vi "Build Common Path Groups.vi"(8 "error in (no error)":errorcluster, 11 "File Group Paths":string[](array[string])) -> (0 "error out":errorcluster, 3 "Common Path map":map{string, string[]}(c390))   [LabVIEW 2019, in "Project.Dependencies Finder.lvlib" / "Dependency Source.lvclass"]
doc: "Order File Group paths in a map by the first folder name. \nThe file name is removed."
uses:
  Dependency Source.lvclass
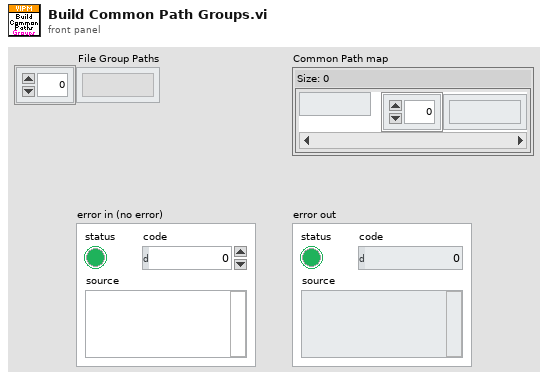
[diagram p1: front panel]
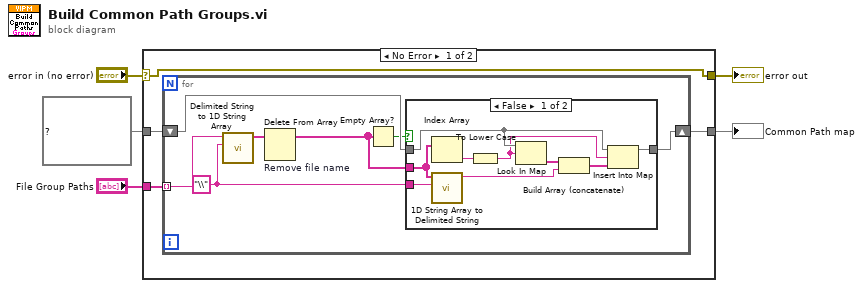
[diagram p0: block diagram]
diagram:
  n1 = case shown="No Error" "error in (no error)" {
    selector: "error in (no error)" -> [w6 w27]
    tunnel: [w6 w27] -> w3
    tunnel: [w9 w28] -> w4
    tunnel: map{string, string[]} {} ("map") -> [w8 w28]
    tunnel: "File Group Paths" -> [w7 _]
    frame No Error {
      n2 = for {
        shift-right: [w16] -> w9
        shift-left: w8 -> [w15]
        tunnel: w7 -> [w14] mode=indexing
        w12 = "\\" ("search string")
        n3 = call <vilib>:"Delimited String to 1D String Array.vi"("delimiter"=w12, "delimited string"=w14) -> ("string array"=w13:string[])  [unwired: 9 in]
        n4 = Delete From Array "Remove file name"(array=w13) -> (array with subset deleted=w11:string[])  [unwired: 2 in, 1 out]
        n5 = Empty Array?(array=w11) -> (empty?=w10:bool)
        n6 = case shown="False" w10 {
          tunnel: [w25 w26] -> w16
          tunnel: w15 -> [w24 w26]
          tunnel: w12 -> [w23 _]
          tunnel: w11 -> [w17 _]
          frame False {
            n7 = Index Array(array=w17) -> (element=w22:string)  [unwired: 1 in]
            n8 = call <vilib>:"1D String Array to Delimited String.vi"("delimiter"=w23, "string array"=w17) -> ("delimited string"=w19:string)  [unwired: 9 in]
            n9 = To Lower Case(string=w22) -> (all lower case string=w21:string)
            n10 = Look In Map(map=w24, key=w21) -> (value=w20:string[])  [unwired: 1 in, 1 out]
            n11 = Build Array (concatenate)(w20, w19) -> (w18:string[])
            n12 = Insert Into Map(map in=w24, key=w21, value=w18) -> (map out=w25:map{string, string[]})  [unwired: 2 out]
          }
          frame True {
          }
        }
      }
    }
    frame Error {
    }
  }
  "Common Path map" <- w4
  "error out" <- w3
